vi "Destroy.vi"(8 "error in (no error)":errorcluster, 11 "Buffer in":refnum<class "Buffer.lvclass">) -> (0 "error out":errorcluster)   [LabVIEW 2020, in "Buffer.lvclass"]
uses:
  Buffer.lvclass
  Buffer.lvclass/Buffer.ctl
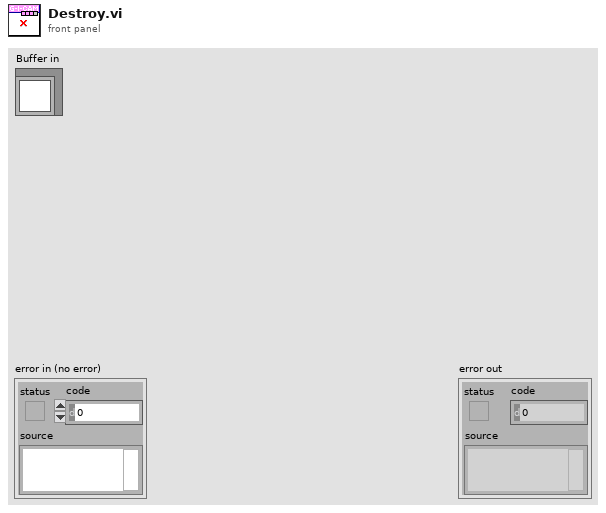
[diagram p1: front panel]
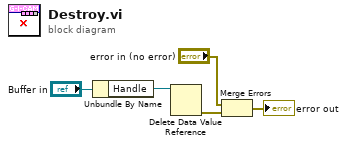
[diagram p0: block diagram]
diagram:
  n1 = Unbundle By Name("Buffer in") -> ("Handle"=w3:refnum<data-value>)
  n2 = Delete Data Value Reference(data value reference=w3) -> (error out=w1:errorcluster)  [unwired: 1 in, 1 out]
  n3 = Merge Errors("error in (no error)", w1) -> (→"error out":errorcluster)
